vi "Display Module - Run Merge Tool.vi"(7 "Calling VI Ref":refnum<vi>) -> ()   [LabVIEW 2020]
panel:
  out "Error":errorcluster
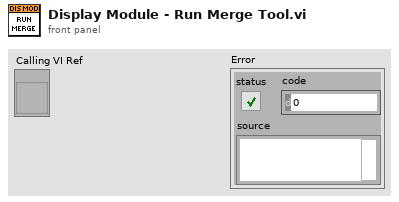
[diagram p1: front panel]
types:
  T1 = enum32{"Bad", "Idle", "Run top level", "Running"}
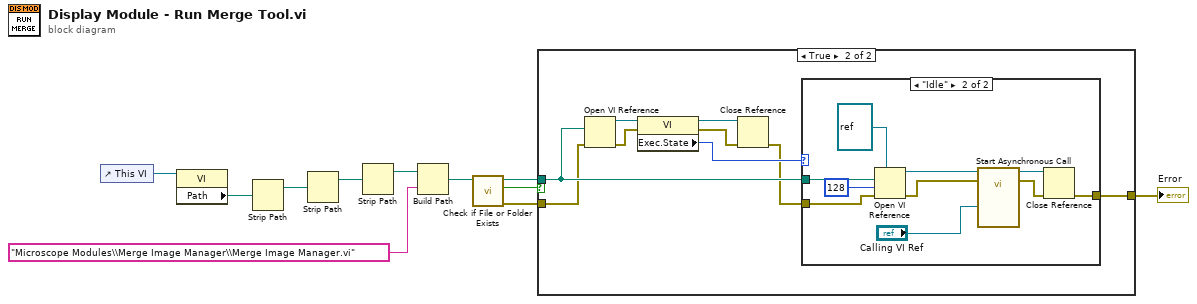
[diagram p0: block diagram]
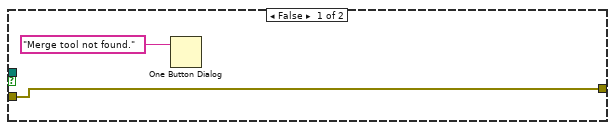
[diagram p2: hidden frame]
diagram:
  n1 = control-ref of="This VI"() -> (w11:refnum<vi>)
  n2 = property class="VI"(reference=w11) -> ("Path"=w10:path)  [unwired: 1 in, 2 out]
  n3 = Strip Path(path=w10) -> (stripped path=w9:path)  [unwired: 1 out]
  n4 = Strip Path(path=w9) -> (stripped path=w2:path)  [unwired: 1 out]
  n5 = Strip Path(path=w2) -> (stripped path=w1:path)  [unwired: 1 out]
  n6 = Build Path(base path=w1, name or relative path="Microscope Modules\\Merge Image Manager\\Merge Image Manager.vi") -> (appended path=w7:path)
  n7 = call <vilib>:"Check if File or Folder Exists.vi"("path"=w7) -> ("error out"=w4:errorcluster, "file or folder exists?"=w6:bool, "dup path"=w5:path)  [unwired: 8 in]
  n8 = case shown="True" w6 {
    tunnel: w5 -> [_ w21]
    tunnel: w4 -> [w12 w19]
    tunnel: [w12 w22] -> w3
    frame False {
      n9 = One Button Dialog(message="Merge tool not found.") -> ()  [unwired: 1 in, 1 out]
    }
    frame True {
      n10 = Open VI Reference(vi path=w21, error in (no error)=w19) -> (vi reference=w20:refnum<vi>, error out=w18:errorcluster)  [unwired: 4 in]
      n11 = property class="VI"(reference=w20, error in=w18) -> (reference out=w17:refnum<vi>, error out=w16:errorcluster, "Exec.State"=w15:T1)
      n12 = Close Reference(reference=w17, error in (no error)=w16) -> (error out=w14:errorcluster)
      n13 = case shown="\"Idle\"" w15 {
        tunnel: w21 -> [_ w33]
        tunnel: w14 -> [w23 w28]
        tunnel: [w23 w27] -> w22
        frame Default {
        }
        frame "Idle" {
          n14 = Open VI Reference(type specifier VI Refnum (for type only)=refnum<vi> refnum, vi path=w33, options=128, error in (no error)=w28) -> (vi reference=w26:refnum<vi>, error out=w24:errorcluster)  [unwired: 2 in]
          n15 = call-by-ref "Start Asynchronous Call"(reference=w26, error in=w24, "Calling VI Ref"="Calling VI Ref") -> (reference out=w30:refnum<vi>, error out=w29:errorcluster)  [unwired: 15 in]
          n16 = Close Reference(reference=w30, error in (no error)=w29) -> (error out=w27:errorcluster)
        }
      }
    }
  }
  "Error" <- w3
